vi "Set Config.vi"(8 "error in (no error)":errorcluster, 10 "Config":T1[](array[typedef]), 11 "DeployResource in":refnum<class "DeployResource.lvclass">) -> (0 "error out":errorcluster, 3 "DeployResource out":refnum<class "DeployResource.lvclass">)   [LabVIEW 2020, in "PicoG-Core.lvlib" / "DeployResource.lvclass"]
uses:
  DeployResource.lvclass
  Config Item.ctl
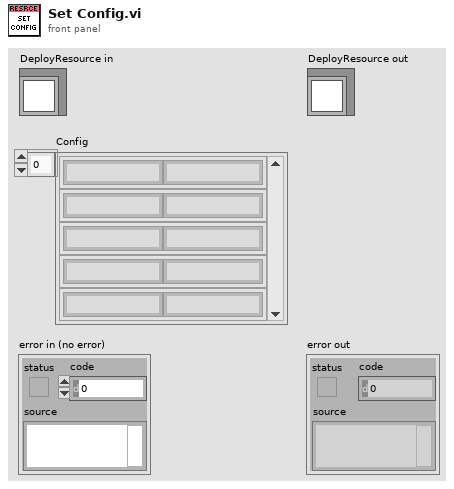
[diagram p1: front panel]
types:
  T1 = typedef "PicoG-Core.lvlib/DeployResource.lvclass/Config Item.ctl" = cluster{"Key":string, "Value":string}
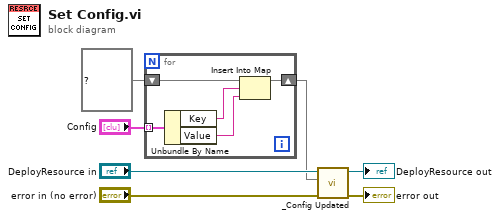
[diagram p0: block diagram]
diagram:
  n1 = for {
    tunnel: "Config" -> [w12] mode=indexing
    shift-right: [w8] -> w1
    shift-left: map{string, string} {} ("map") -> [w11]
    n2 = Unbundle By Name(w12) -> ("Key"=w10:string, "Value"=w9:string)
    n3 = Insert Into Map(map in=w11, key=w10, value=w9) -> (map out=w8:map{string, string})  [unwired: 2 out]
  }
  n4 = call-dynamic "_Config Updated.vi"("error in (no error)"="error in (no error)", "Config Map"=w1, "DeployResource in"="DeployResource in") -> ("error out"=→"error out":errorcluster, "DeployResource out"=→"DeployResource out":refnum<class "DeployResource.lvclass">)  [unwired: 7 in]
